vi "ShooterCam.vi"(1 "trigger":bool) -> ()   [LabVIEW 2012]
uses:
  Robot Global Data.vi
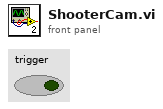
[diagram p1: front panel]
types:
  T1 = typedef "WPI_DigitalInputDevRef.ctl" = cluster{"DevStatus":errorcluster, "DIO Channel":T2, "Digital Module":T3}
  T2 = typedef "FPGA_DIOChannel.ctl" = enum8{"DIO 1", "DIO 2", "DIO 3", "DIO 4", "DIO 5", "DIO 6", "DIO 7", "DIO 8", "DIO 9", "DIO 10", "DIO 11", "DIO 12", "DIO 13", "DIO 14", "Invalid"}
  T3 = typedef "FPGA_TypedefDigitalModule.ctl" = enum16{"Digital Module 1", "Digital Module 2"}
  T4 = typedef "WPI_MotorControlDeviceRef.ctl" = cluster{"DeviceStatus":errorcluster, "Type":enum16{"PWM", "CAN"}, "PWM":cluster{"Digital Module":T3, "PWM Channel":T5, "DeadBand":T6}, "CAN":cluster{"Device Number":u8, "Control Mode":T7, "Semaphore":T8, "Max Vout":dbl}, "Invert":bool, "TransformRef":T9, "InvTransformRef":T9}
  T5 = typedef "FPGA_DIOPWMChannel.ctl" = enum8{"PWM 1", "PWM 2", "PWM 3", "PWM 4", "PWM 5", "PWM 6", "PWM 7", "PWM 8", "PWM 9", "PWM 10", "Invalid"}
  T6 = typedef "WPI_PWMDeadband.ctl" = cluster{"Name":string, "maxPositivePwm":i32, "minPositivePwm":i32, "centerPwm":i32, "maxNegativePwm":i32, "minNegativePwm":i32, "angularRange":u16}
  T7 = typedef "WPI_CANJaguar_ControlMode.ctl" = enum8{"Percent VBus", "Current", "Speed", "Position", "Voltage"}
  T8 = typedef "Semaphore RefNum" = refnum<k1>
  T9 = typedef "WPI_PWMTransform_ConPane.ctl" = refnum<vi>
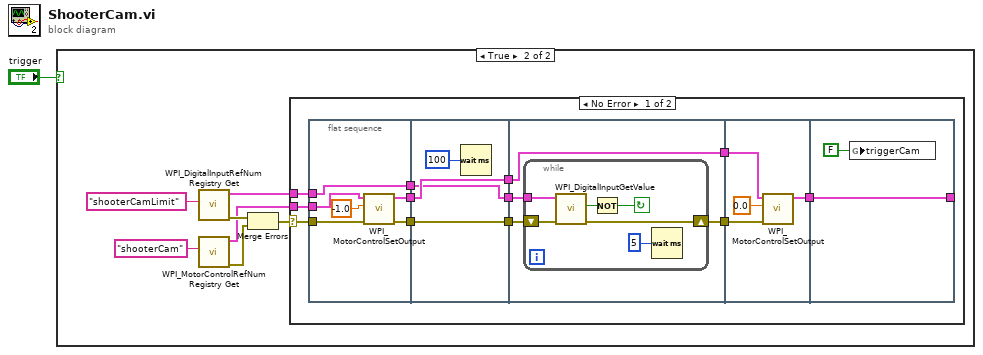
[diagram p0: block diagram]
diagram:
  n1 = case shown="True" "trigger" {
    frame False {
    }
    frame True {
      n2 = call <vilib>:"WPI_DigitalInputRefNum Registry Get.vi"("refnum name"="shooterCamLimit") -> ("error out"=w6:errorcluster, "DigitalInputDevRef"=w3:T1)  [unwired: 9 in]
      n3 = call <vilib>:"WPI_MotorControlRefNum Registry Get.vi"("refnum name"="shooterCam") -> ("error out"=w5:errorcluster, "MotorControlDevRef"=w2:T4)  [unwired: 9 in]
      n4 = Merge Errors(w6, w5) -> (w4:errorcluster)
      n5 = case shown="No Error" w4 {
        selector: w4 -> [w19 _]
        tunnel: w3 -> [w16 _]
        tunnel: w2 -> [w20 _]
        frame No Error {
          n6 = flat-sequence {
            tunnel: w20 -> [w26]
            tunnel: w19 -> [w24]
            tunnel: [w23] -> w14
            tunnel: [w22] -> w12
            tunnel: [w21] -> w10
            tunnel: w16 -> [w21]
            tunnel: w14 -> [w30]
            tunnel: [w30] -> w13
            tunnel: w12 -> [w29]
            tunnel: [w29] -> w11
            tunnel: w10 -> [w28]
            tunnel: [w28] -> w9
            tunnel: w13 -> [w32]
            tunnel: w11 -> [w34]
            tunnel: [w32] -> w18
            tunnel: [w33] -> w17
            tunnel: w9 -> [w31]
            tunnel: w18 -> [w43]
            tunnel: w17 -> [w41]
            tunnel: [w42] -> w15
            tunnel: [w46] -> _
            tunnel: w15 -> [w46]
            frame #0 {
              n7 = call <vilib>:"WPI_MotorControlSetOutput.vi"("error in (no error)"=w24, "Output"=-1.0, "MotorControlDevRef"=w26) -> ("error out"=w22:errorcluster, "MotorControlDevRef"=w23:T4)  [unwired: 6 in, 1 out]
            }
            frame #1 {
              n8 = Wait (ms)(milliseconds to wait=u32 100) -> ()  [unwired: 1 out]
            }
            frame #2 {
              n9 = while {
                shift-right: [w36] -> w33
                shift-left: w34 -> [w40]
                tunnel: w31 -> [w35]
                stop <- w38 continue-if-true
                n10 = call <vilib>:"WPI_DigitalInputGetValue.vi"("error in (no error)"=w40, "DigitalInputDevRef"=w35) -> ("error out"=w36:errorcluster, "Value"=w39:bool)  [unwired: 7 in, 1 out]
                n11 = Not(x=w39) -> (.not. x?=w38:bool)
                n12 = Wait (ms)(milliseconds to wait=u32 5) -> ()  [unwired: 1 out]
              }
            }
            frame #3 {
              n13 = call <vilib>:"WPI_MotorControlSetOutput.vi"("error in (no error)"=w41, "Output"=0.0, "MotorControlDevRef"=w43) -> ("MotorControlDevRef"=w42:T4)  [unwired: 6 in, 2 out]
            }
            frame #4 {
              n14 = global write "Robot Global Data.vi" "triggerCam"(FALSE ("triggerCam")) -> ()
            }
          }
        }
        frame Error {
        }
      }
    }
  }
